vi "Remote robot control (robot acquires video).vi"() -> ()   [LabVIEW 2012]
doc: "Main VI that runs on the host for teleoperation. This VI sends teleop commands to the robot via UDP and receives video back from the robot using network streams."
uses:
  Teleop command.ctl
  Safety commands.ctl
  Robot globals (robot acquires video).vi
  Host globals (robot acquires video).vi
  <vilib>/Utility/inputDevices.llb/closeKeyboard.vi
  Convert keyboard to teleop command.vi
panel:
  out "error out":errorcluster
  in  "Robot IP address":string="XXX.XXX.XXX.XXX"
  in  "Stop":bool
  out "Current teleop command":T1
  out "Robot video feed":T2(plugin-control)
  # "Change Robot IP address to match the IP address of the robot you are controlling (Robot should be running \"Robot main.vi\")"
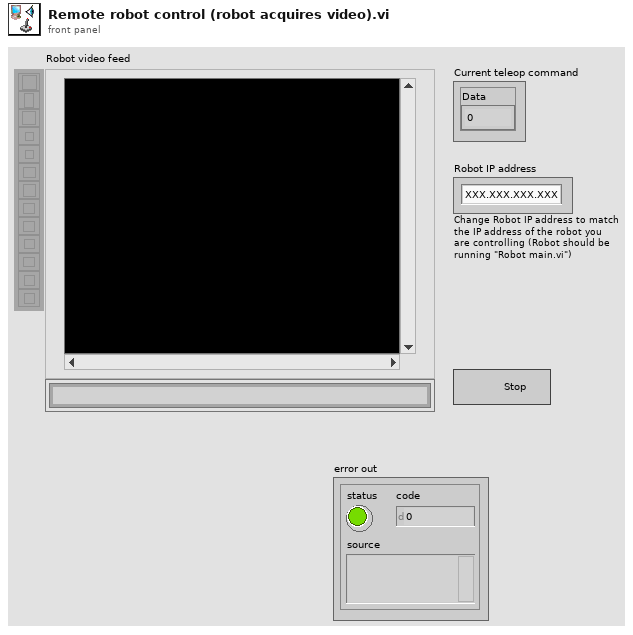
[diagram p1: front panel]
types:
  T1 = typedef "Teleop command.ctl" = cluster{"Data":dbl}
  T2 = typedef "IMAQ Image.ctl" = refnum<image>
  T3 = typedef "Safety commands.ctl" = cluster{"Stop":bool, "Pause":bool}
  T4 = typedef "Image Type" = u32
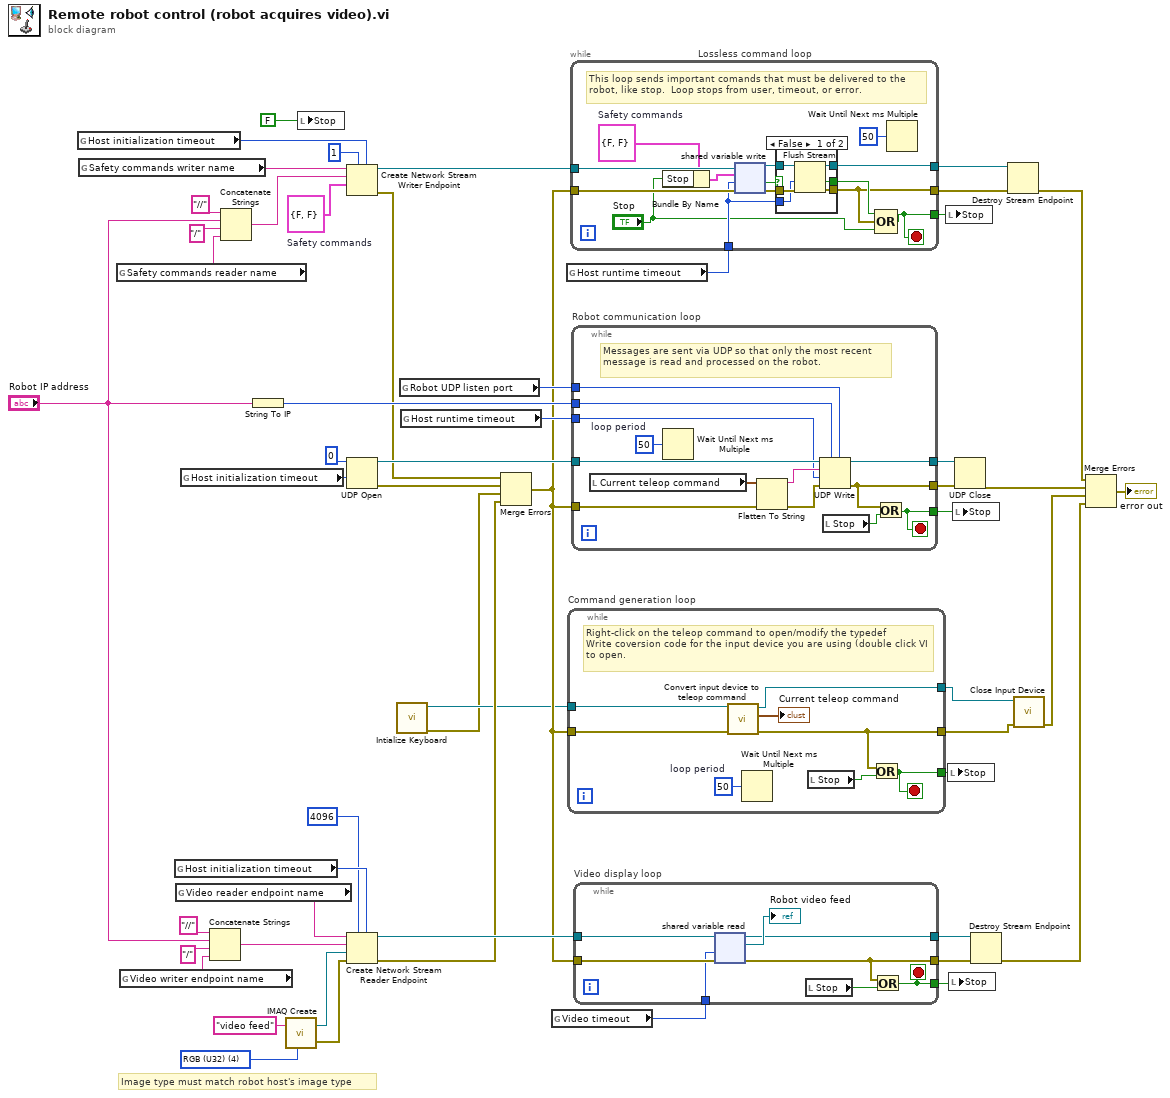
[diagram p0: block diagram]
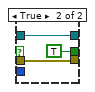
[diagram p2: hidden frame]
diagram:
  w18 = T3 {"Stop"=FALSE, "Pause"=FALSE}  # Safety commands
  w54 = T4 4 items=["Grayscale (U8)", "Grayscale (I16)", "Grayscale (SGL)", "Complex (CSG)", "RGB (U32)", "HSL (U32)", "RGB (U64)", "Grayscale (U16)"] ("Image Type")
  # "Image type must match robot host's image type"
  n1 = global read "Host globals (robot acquires video).vi" "Host initialization timeout"() -> (w10:i32)
  n2 = global read "Host globals (robot acquires video).vi" "Safety commands writer name"() -> (w16:string)
  n3 = global read "Robot globals (robot acquires video).vi" "Safety commands reader name"() -> (w4:string)
  n4 = global read "Robot globals (robot acquires video).vi" "Video writer endpoint name"() -> (w33:string)
  n5 = global read "Host globals (robot acquires video).vi" "Host initialization timeout"() -> (w37:i32)
  n6 = global read "Host globals (robot acquires video).vi" "Video reader endpoint name"() -> (w28:string)
  n7 = global read "Host globals (robot acquires video).vi" "Host initialization timeout"() -> (w20:i32)
  n8 = Concatenate Strings("//" ("string"), "Robot IP address", "/" ("string"), w33) -> (w30:string)
  n9 = Concatenate Strings("//" ("string"), "Robot IP address", "/" ("string"), w4) -> (w17:string)
  n10 = String To IP(1:"Robot IP address") -> (0:w38:u32)
  n11 = call "IMAQ Create"("Image Name"="video feed", "Image Type"=w54) -> ("New Image"=w53:T2, "error out"=w48:errorcluster)  [unwired: 3 in]
  n12 = local write "Stop"(FALSE ("Stop")) -> ()
  n13 = Create Network Stream Writer Endpoint(5:w10, 7:1 ("writer buffer size"), 9:w18, 10:w17, 11:w16) -> (0:w12:errorcluster, 3:w25:refnum<k21>)  [unwired: 2 in]
  n14 = UDP Open(9:w20, 11:u16 0 ("port")) -> (port=w47:refnum<k16>, 0:w13:errorcluster)  [unwired: 3 in, 1 out]
  n15 = Create Network Stream Reader Endpoint(5:w37, 7:4096 ("reader buffer size"), 8:w48, 9:w53, 10:w30, 11:w28) -> (0:w8:errorcluster, 3:w52:refnum<k21>)  [unwired: 1 in]
  n16 = call <vilib>:"Intialize Keyboard.vi"() -> ("error out"=w2:errorcluster, "device ID"=w3:refnum<k1>)  [unwired: 10 in]
  n17 = global read "Robot globals (robot acquires video).vi" "Robot UDP listen port"() -> (w39:u16)
  n18 = global read "Host globals (robot acquires video).vi" "Host runtime timeout"() -> (w29:i32)
  n19 = Merge Errors(w12, w13, w2, w8) -> (w9:errorcluster)
  n20 = global read "Robot globals (robot acquires video).vi" "Video timeout"() -> (w36:i32)
  n21 = global read "Host globals (robot acquires video).vi" "Host runtime timeout"() -> (w19:i32)
  n22 = while "Command generation loop" {
    tunnel: [w62] -> w42
    tunnel: [w57] -> w41
    tunnel: [w60] -> w40
    tunnel: w9 -> [w58]
    tunnel: w3 -> [w55]
    stop <- w62 stop-if-true
    w59 = u32 50  # loop period
    # "Right-click on the teleop command to open/modify the typedef\nWrite coversion code for the input device you are using (double click VI to open."
    n23 = call-poly "Convert input device to teleop command.vi"("error in (no error)"=w58, "Keyboard in"=w55) -> ("error out"=w57:errorcluster, "Teleop command out"=→"Current teleop command":T1, "Keyboard out"=w60:refnum<k1>)  [unwired: 7 in]
    n24 = Wait Until Next ms Multiple(millisecond multiple=w59) -> ()  [unwired: 1 out]
    n25 = local read "Stop"() -> (w56:bool)
    n26 = Or(x=w57, y=w56) -> (x .or. y?=w62:bool)
  }
  n27 = while "Lossless command loop" {
    tunnel: [w66] -> w26
    tunnel: w9 -> [w76]
    tunnel: w25 -> [w75]
    tunnel: [w70] -> w24
    tunnel: [w65] -> w23
    tunnel: w19 -> [w69]
    stop <- w66 stop-if-true
    w74 = T3 {"Stop"=FALSE, "Pause"=FALSE}  # Safety commands
    # "This loop sends important comands that must be delivered to the robot, like stop.  Loop stops from user, timeout, or error."
    n28 = Bundle By Name(cluster=w74, "Stop"="Stop") -> (w73:T3)
    n29 = shared-variable-write(w75, w76, w73, w69) -> (w71:refnum<k21>, w72:errorcluster, w68:bool)
    n30 = case shown="False" w68 {
      tunnel: w72 -> [w82 w84]
      tunnel: w71 -> [w81 w85]
      tunnel: [w80 w85] -> w70
      tunnel: [w79 w84] -> w65
      tunnel: w69 -> [w78 _]
      tunnel: [w77 TRUE ("timed out?")] -> w67
      frame False {
        n31 = Flush Stream(8:w82, 9:w78, 11:w81) -> (0:w79:errorcluster, 1:w77:bool, 3:w80:refnum<k21>)  [unwired: 1 in]
      }
      frame True {
      }
    }
    n32 = Compound Arithmetic op=OR(w67, w65, "Stop") -> (w66:bool)
    n33 = Wait Until Next ms Multiple(millisecond multiple=u32 50) -> ()  [unwired: 1 out]
  }
  n34 = while "Robot communication loop" {
    tunnel: w47 -> [w95]
    tunnel: w9 -> [w97]
    tunnel: [w94] -> w46
    tunnel: [w91] -> w45
    tunnel: [w90] -> w43
    tunnel: w39 -> [w89]
    tunnel: w38 -> [w88]
    tunnel: w29 -> [w87]
    stop <- w90 stop-if-true
    w86 = u32 50  # loop period
    # "Messages are sent via UDP so that only the most recent message is read and processed on the robot."
    n35 = local read "Current teleop command"() -> (w98:T1)
    n36 = Wait Until Next ms Multiple(millisecond multiple=w86) -> ()  [unwired: 1 out]
    n37 = Flatten To String(anything=w98, error in (no error)=w97) -> (data string=w96:string, error out=w93:errorcluster)  [unwired: 2 in, 1 out]
    n38 = UDP Write(address=w88, port or service name=w89, connection ID=w95, data in=w96, 8:w93, 9:w87) -> (error out=w91:errorcluster, 3:w94:refnum<k16>)
    n39 = local read "Stop"() -> (w92:bool)
    n40 = Or(x=w91, y=w92) -> (x .or. y?=w90:bool)
  }
  n41 = while "Video display loop" {
    tunnel: w52 -> [w106]
    tunnel: w9 -> [w104]
    tunnel: [w103] -> w51
    tunnel: [w100] -> w50
    tunnel: [w101] -> w44
    tunnel: w36 -> [w99]
    stop <- w101 stop-if-true
    n42 = shared-variable-read(w106, w104, w99) -> (w103:refnum<k21>, w100:errorcluster, →"Robot video feed":T2)  [unwired: 1 out]
    n43 = local read "Stop"() -> (w102:bool)
    n44 = Or(x=w100, y=w102) -> (x .or. y?=w101:bool)
  }
  n45 = local write "Stop"(w26) -> ()
  n46 = local write "Stop"(w42) -> ()
  n47 = local write "Stop"(w44) -> ()
  n48 = local write "Stop"(w43) -> ()
  n49 = UDP Close(connection ID=w46, 8:w45) -> (error out=w34:errorcluster)  [unwired: 1 out]
  n50 = Destroy Stream Endpoint(8:w50, 11:w51) -> (0:w27:errorcluster)
  n51 = Destroy Stream Endpoint(8:w23, 11:w24) -> (0:w15:errorcluster)
  n52 = call-poly <vilib>:"Close Input Device.vi"("error in (no error)"=w41, "device ID"=w40) -> ("error out"=w35:errorcluster)  [unwired: 8 in]
  n53 = Merge Errors(w15, w34, w35, w27) -> (→"error out":errorcluster)
